vi "参考-报表颜色.vi"(4 "列":i8, 5 "行":i8, 6 "下限":dbl, 7 "上限":dbl, 8 "error in (no error)":errorcluster caption="错误输入（无错误）", 9 "table index (-1)":i16=-1, 10 "厚度值":dbl, 11 "report in":refnum<class "NI_report.lvclass"> caption="报表输入") -> (0 "error out":errorcluster caption="错误输出", 3 "report out":refnum<class "NI_report.lvclass"> caption="报表输出")   [LabVIEW 2018]
uses:
  <vilib>/Utility/NIReport.llb/NI_report.lvclass
  <vilib>/Utility/NIReport.llb/Word/NI_Word.lvclass
  <vilib>/addons/_office/NI_ReportGenerationToolkit.lvlib
panel:
  out "范围内？":bool
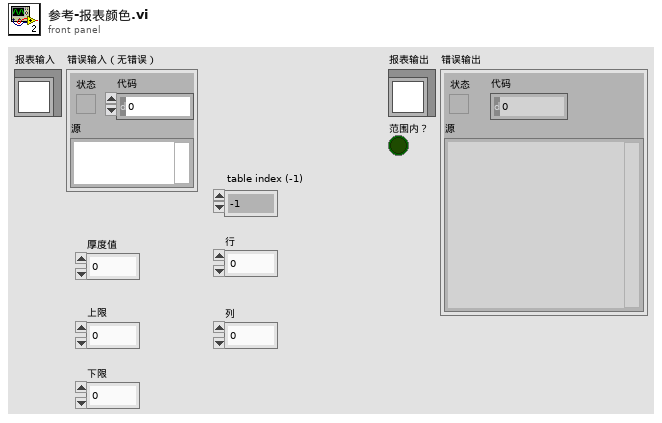
[diagram p1: front panel]
types:
  T1 = cluster{"OutsideLineStyle":i32, "OutsideColor":i32, "OutsideLineWidth":i32, "InsideLineStyle":i32, "InsideColor":i32, "InsideLineWidth":i32, "BackgroundPatternColor":i32}
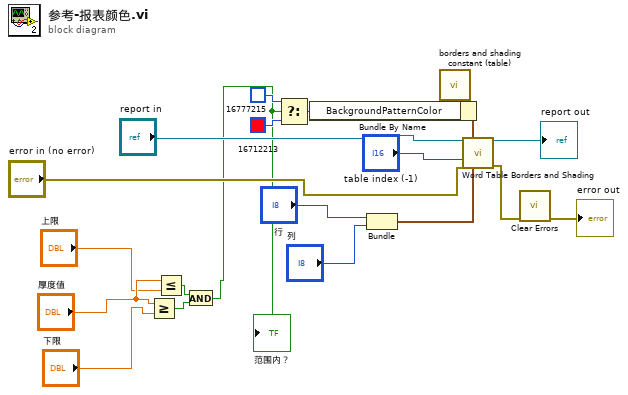
[diagram p0: block diagram]
diagram:
  n1 = Greater Or Equal?(x="厚度值", y="下限") -> (x >= y?=w2:bool)
  n2 = Less Or Equal?(x="厚度值", y="上限") -> (x <= y?=w3:bool)
  n3 = And(x=w3, y=w2) -> (x .and. y?=w1:bool)
  "范围内？" <- w1
  n4 = Select(t=u32 16777215, s=w1, f=u32 16712213) -> (s? t:f=w15:u32)
  n5 = Bundle("行"="行", "列"="列") -> (w18:cluster{"行":i8, "列":i8})  [unwired: 1 in]
  n6 = call <vilib>:"borders and shading constant (table).vi"() -> ("borders and shading"=w20:T1)
  n7 = Bundle By Name(cluster=w20, "BackgroundPatternColor"=w15) -> (w19:T1)
  n8 = call <vilib>:"Word Table Borders and Shading.vi"("report in"="report in", "borders and shading"=w19, "table index (-1)"="table index (-1)", "error in (no error)"="error in (no error)", "start (-1, -1)"=w18) -> ("report out"=→"report out":refnum<class "NI_report.lvclass">, "error out"=w8:errorcluster)  [unwired: 9 in]
  n9 = call <vilib>:"Clear Errors.vi"("error in (no error)"=w8) -> ("error out"=→"error out":errorcluster)  [unwired: 5 in, 1 out]
